vi "rename dialog.vi"(11 "module editor node in":refnum<class "module editor node.lvclass">) -> (2 "changed":bool, 3 "module editor node out":refnum<class "module editor node.lvclass">)   [LabVIEW 2013, in "PL Framework Configuration Tool.lvlib" / "module editor node.lvclass"]
uses:
  module editor node.lvclass
  <vilib>/NI/Configuration Framework/serializable configuration/get alias.vi
  <vilib>/NI/Configuration Framework/serializable configuration/set alias.vi
  <vilib>/NI/Configuration Framework/serializable configuration/NISE_CEF_serializable configuration.lvclass
panel:
  in  "cancel":bool
  in  "commit":bool
  in  "New Alias":string
  out "Current Alias":string
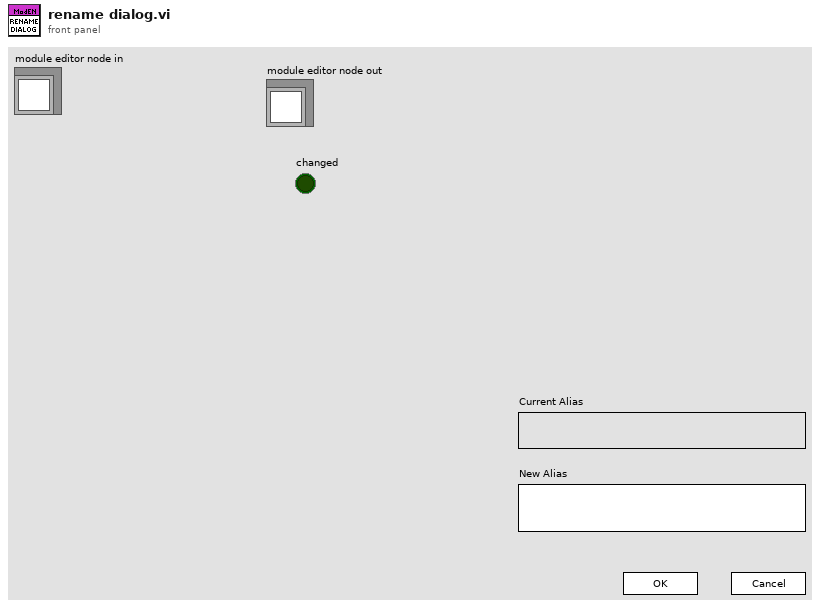
[diagram p1: front panel]
types:
  T1 = enum8{"Enabled", "Disabled", "Disabled and Grayed Out"}
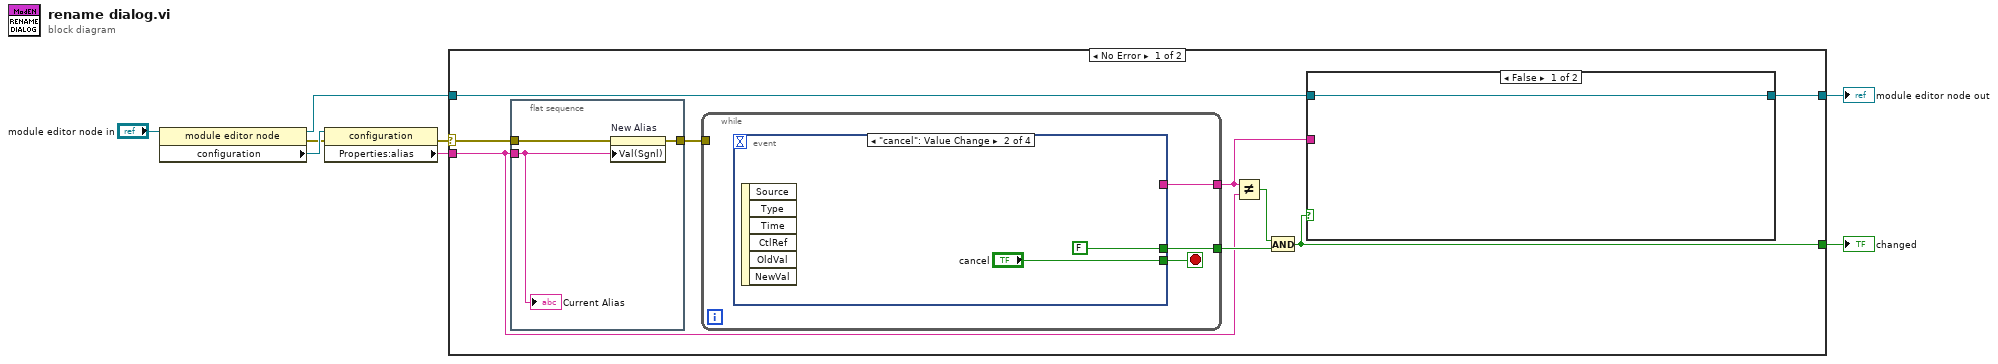
[diagram p0: block diagram]
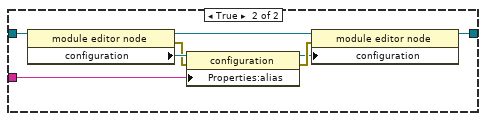
[diagram p2: hidden frame]
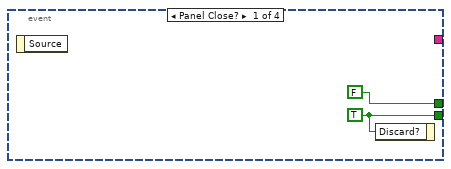
[diagram p3: hidden frame]
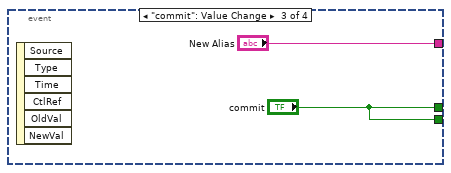
[diagram p4: hidden frame]
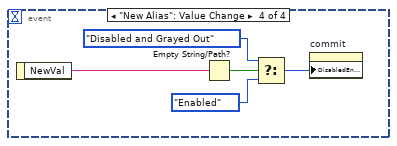
[diagram p5: hidden frame]
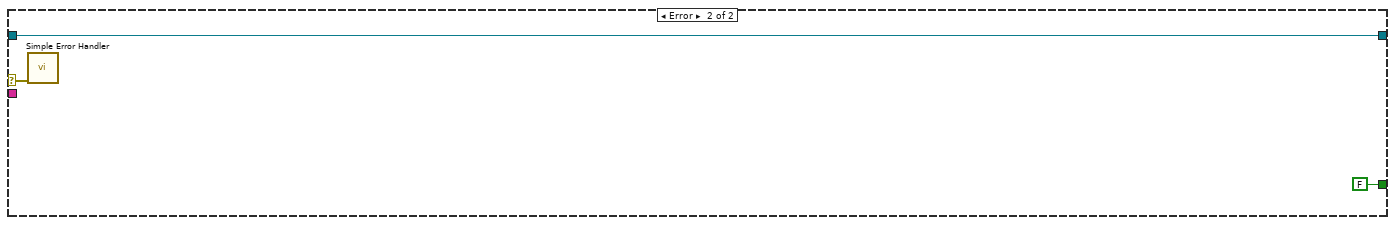
[diagram p6: hidden frame]
diagram:
  n1 = property class="module editor node"(reference="module editor node in") -> (reference out=w3:refnum<class "module editor node.lvclass">, error out=w6:errorcluster, "configuration"=w7:refnum<class "NISE_CEF_serializable configuration.lvclass">)  [unwired: 1 in]
  n2 = property class="configuration"(reference=w7, error in=w6) -> (error out=w5:errorcluster, "Properties:alias"=w1:string)  [unwired: 1 out]
  n3 = case shown="No Error" w5 {
    selector: w5 -> [w16 w46]
    tunnel: [w14 w45] -> w4
    tunnel: w3 -> [w13 w45]
    tunnel: [w12 FALSE] -> w2
    tunnel: w1 -> [w10 _]
    frame No Error {
      n4 = flat-sequence {
        tunnel: w10 -> [w43]
        tunnel: [w41] -> w17
        tunnel: w16 -> [w42]
        frame #0 {
          n5 = property on="New Alias" class="Str"(error in=w42, "Val(Sgnl)"=w43) -> (error out=w41:errorcluster)  [unwired: 1 in, 1 out]
          "Current Alias" <- w43
        }
      }
      n6 = while {
        tunnel: w17 -> [_]
        tunnel: [w29] -> w15
        tunnel: [w27] -> w9
        stop <- w28 stop-if-true
        n7 = event shown="[1] \"cancel\": Value Change" {
          selector: _ -> [_ _ _ _]
          dyn-events: _ -> [_ _ _ _]
          timeout: _ -> [_ _ _ _]
          tunnel: [FALSE FALSE "commit" _] -> w29
          tunnel: [w30 "cancel" "commit" _] -> w28
          tunnel: [_ _ "New Alias" _] -> w27
          event Panel Close? {
            w30 = TRUE ("Discard?")
            n8 = event-data() -> ()  [unwired: 1 in, 1 out]
            n9 = event-data("Discard?"=w30) -> ()  [unwired: 1 in, 1 out]
          }
          event "cancel": Value Change {
            n10 = event-data() -> ()  [unwired: 1 in, 6 out]
          }
          event "commit": Value Change {
            n11 = event-data() -> ()  [unwired: 1 in, 6 out]
          }
          event "New Alias": Value Change {
            n12 = event-data() -> ("NewVal"=w37:string)  [unwired: 1 in]
            n13 = Empty String/Path?(string/path=w37) -> (empty?=w36:bool)
            n14 = Select(t=T1."Disabled and Grayed Out" ("Disabled"), s=w36, f=T1."Enabled" ("Disabled")) -> (s? t:f=w40:T1)
            n15 = property on="commit" class="Bool"("DisabledEnum"=w40) -> ()  [unwired: 2 in, 2 out]
          }
        }
      }
      n16 = Not Equal?(x=w9, y=w10) -> (x != y?=w11:bool)
      n17 = And(x=w11, y=w15) -> (x .and. y?=w12:bool)
      n18 = case shown="False" w12 {
        tunnel: [w18 w24] -> w14
        tunnel: w13 -> [w18 w26]
        tunnel: w9 -> [_ w19]
        frame False {
        }
        frame True {
          n19 = property class="module editor node"(reference=w26) -> (reference out=w25:refnum<class "module editor node.lvclass">, error out=w22:errorcluster, "configuration"=w23:refnum<class "NISE_CEF_serializable configuration.lvclass">)  [unwired: 1 in]
          n20 = property class="configuration"(reference=w23, error in=w22, "Properties:alias"=w19) -> (reference out=w20:refnum<class "NISE_CEF_serializable configuration.lvclass">, error out=w21:errorcluster)
          n21 = property class="module editor node"(reference=w25, error in=w21, "configuration"=w20) -> (reference out=w24:refnum<class "module editor node.lvclass">)  [unwired: 1 out]
        }
      }
    }
    frame Error {
      n22 = call <vilib>:"Simple Error Handler.vi"("error in (no error)"=w46) -> ()  [unwired: 4 in, 5 out]
    }
  }
  "module editor node out" <- w4
  "changed" <- w2
